vi "Create Dot.vi"(7 "3D Scatter Property":T4={"General Property"={"Plot Name"="", "Coordinate System"=enum."Cartesian", "Opacity"=0.0}, "Projection Property"={"Draw XY"=FALSE, "Draw YZ"=FALSE, "Draw XZ"=FALSE}, "Plot Property"={"Sprite Type"=enum."Empty Square", "Point Size"=0.0, "Color Ramp Cluster"={"Color Ramp Style"=enum."None", "Color Ramp Array"=[16711934, 393471, 57855, 4390754, 16449346, 16744722, 16711680], "Color Ramp Index"=[45, 91, 133, 175, 219, 255], "Interpolate?"=FALSE, "Logarithm?"=FALSE}}}, 8 "error in (no error)":errorcluster, 9 "Actual Transform In":T7, 10 "Plot Representation In":T1, 11 "Plot Object In":refnum<vi>) -> (0 "error out":errorcluster, 1 "Actual Transform Out":T7, 2 "Plot Representation Out":T1, 3 "Plot Object Out":refnum<vi>, 4 "Dot Object Out":refnum<vi>)   [LabVIEW 2020, in "3D Scatter.lvclass"]
uses:
  <vilib>/Math Plots/3D Math Plots/3D Scatter/3D Scatter/3D Scatter.lvclass
  <vilib>/Math Plots/3D Math Plots/3D Plot/3D Plot/Typedef/Actual Transform.ctl
  <vilib>/Math Plots/3D Math Plots/3D Plot/3D Plot/Typedef/Range Clusters.ctl
  <vilib>/Math Plots/3D Math Plots/3D Plot/3D Plot/Typedef/Plot Representation.ctl
  <vilib>/Math Plots/3D Math Plots/3D Plot/3D Plot/Typedef/Mesh Data.ctl
  <vilib>/Math Plots/3D Math Plots/3D Scatter/3D Scatter/Typedef/3D Scatter Property.ctl
  <vilib>/Math Plots/3D Math Plots/3D Plot/3D Plot/Typedef/Sprite Type.ctl
  <vilib>/Math Plots/3D Math Plots/3D Plot/3D Plot/Typedef/Color Ramp Cluster.ctl
  <vilib>/picture/3D Picture Control/NI_3D Picture Control.lvlib
  <vilib>/Math Plots/3D Math Plots/3D Plot/3D Plot/3D Plot.lvclass
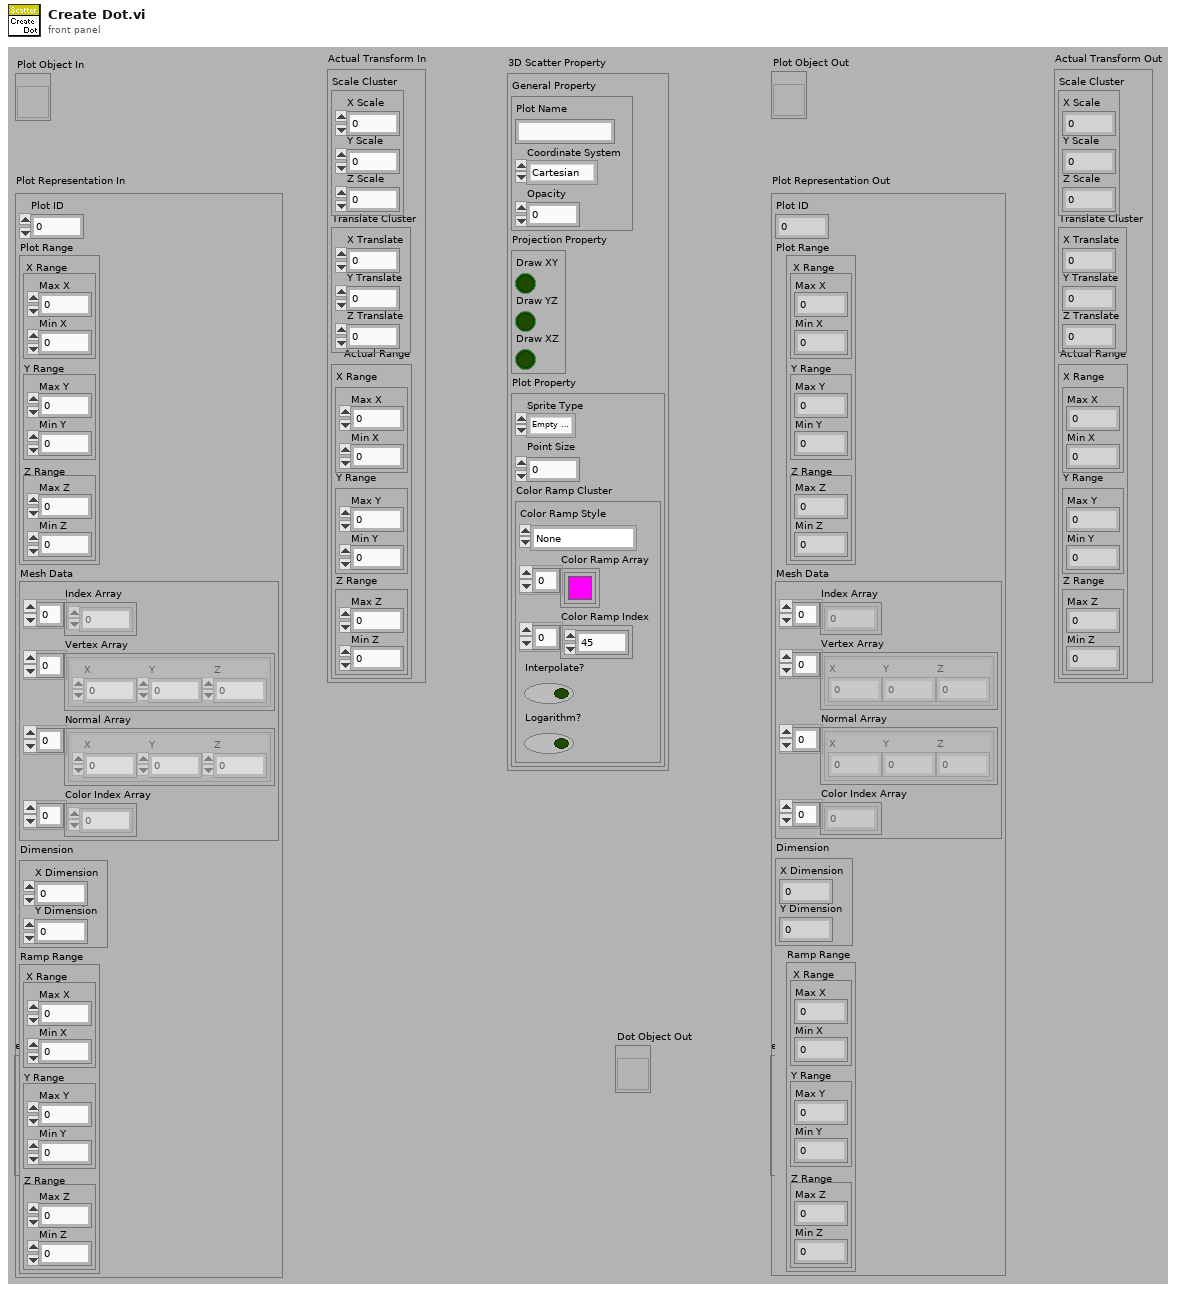
[diagram p1: front panel]
types:
  T1 = typedef "3D Plot.lvclass/Plot Representation.ctl" = cluster{"Plot ID":i32, "Plot Range":T2, "Mesh Data":T3, "Dimension":cluster{"X Dimension":i32, "Y Dimension":i32}, "Ramp Range":T2}
  T2 = typedef "3D Plot.lvclass/Range Clusters.ctl" = cluster{"X Range":cluster{"Max X":sgl, "Min X":sgl}, "Y Range":cluster{"Max Y":sgl, "Min Y":sgl}, "Z Range":cluster{"Max Z":sgl, "Min Z":sgl}}
  T3 = typedef "3D Plot.lvclass/Mesh Data.ctl" = cluster{"Index Array":u32[], "Vertex Array":cluster{"X":sgl, "Y":sgl, "Z":sgl}[], "Normal Array":cluster{"X":sgl, "Y":sgl, "Z":sgl}[], "Color Index Array":i32[]}
  T4 = typedef "3D Scatter.lvclass/3D Scatter Property.ctl" = cluster{"General Property":cluster{"Plot Name":string, "Coordinate System":enum16{"Cartesian", "Cylindrical", "Spherical"}, "Opacity":sgl}, "Projection Property":cluster{"Draw XY":bool, "Draw YZ":bool, "Draw XZ":bool}, "Plot Property":cluster{"Sprite Type":T5, "Point Size":sgl, "Color Ramp Cluster":T6}}
  T5 = typedef "3D Plot.lvclass/Sprite Type.ctl" = enum16{"None", "Empty Square", "Solid Square", "Empty Diamond", "Solid Diamond", "Empty Circle", "Solid Circle", "Asterisk", "Bold X", "Wireframe Sphere", "Solid Sphere", "Wireframe Cube", "Solid Cube"}
  T6 = typedef "3D Plot.lvclass/Color Ramp Cluster.ctl" = cluster{"Color Ramp Style":enum16{"None", "Shaded", "Color spectrum", "Grey scale", "Custom"}, "Color Ramp Array":u32[], "Color Ramp Index":i32[], "Interpolate?":bool, "Logarithm?":bool}
  T7 = typedef "3D Plot.lvclass/Actual Transform.ctl" = cluster{"Scale Cluster":cluster{"X Scale":sgl, "Y Scale":sgl, "Z Scale":sgl}, "Translate Cluster":cluster{"X Translate":sgl, "Y Translate":sgl, "Z Translate":sgl}, "Actual Range":T2}
  T8 = enum16{"Points", "Lines", "Line Strip", "Line Loop", "Triangles", "Triangle Strip", "Triangle Fan", "Quads", "Quad Strip", "Polygon"}
  T9 = enum16{"Overall", "Per Primitive", "Per Vertex", "Binding Off"}
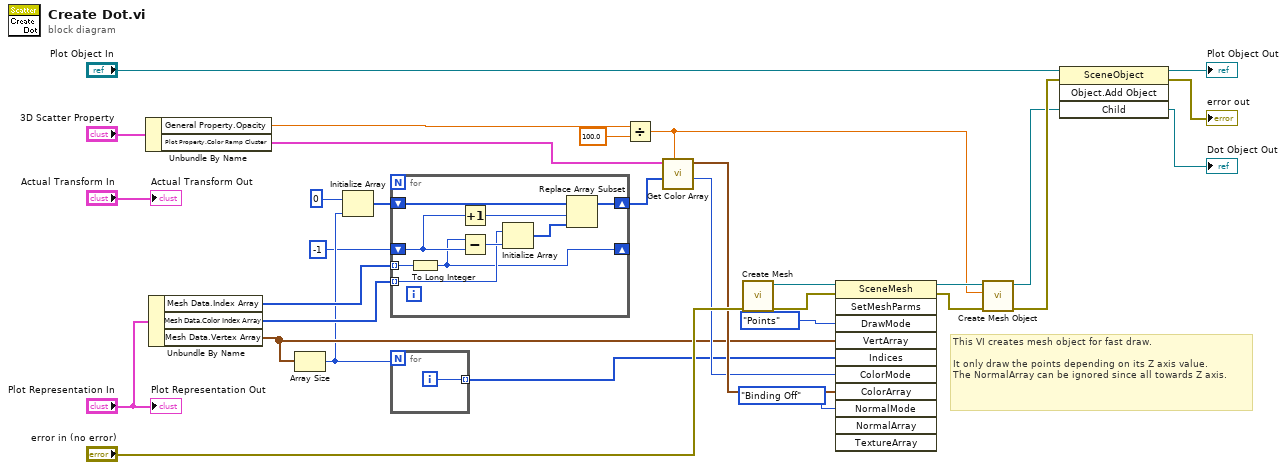
[diagram p0: block diagram]
diagram:
  # "This VI creates mesh object for fast draw.\n\nIt only draw the points depending on its Z axis value. \nThe NormalArray can be ignored since all towards Z axis."
  n1 = Unbundle By Name("3D Scatter Property") -> ("General Property.Opacity"=w24:sgl, "Plot Property.Color Ramp Cluster"=w10:T6)
  n2 = Unbundle By Name("Plot Representation In") -> ("Mesh Data.Index Array"=w8:u32[], "Mesh Data.Color Index Array"=w7:i32[], "Mesh Data.Vertex Array"=w6:cluster{"X":sgl, "Y":sgl, "Z":sgl}[])
  n3 = Array Size(array=w6) -> (size(s)=w5:i32)
  n4 = Initialize Array(0, w5) -> (w4:i32[])
  n5 = for {
    tunnel: w8 -> [w34] mode=indexing
    tunnel: w7 -> [w39] mode=indexing
    shift-right: [w37] -> w3
    shift-left: w4 -> [w38]
    shift-right: [w33] -> _
    shift-left: -1 -> [w35]
    n6 = To Long Integer(number=w34) -> (32bit integer=w33:i32)
    n7 = Increment(x=w35) -> (x+1=w32:i32)
    n8 = Subtract(x=w33, y=w35) -> (x-y=w40:i32)
    n9 = Initialize Array(w39, w40) -> (w36:i32[])
    n10 = Replace Array Subset(array=w38, new element=w36, index=w32) -> (w37:i32[])
  }
  n11 = for {
    N: w5 -> [_]
    tunnel: [w41] -> w9 mode=indexing
    i -> [w41]
  }
  n12 = Divide(x=w24, y=sgl 100.0) -> (x/y=w11:sgl)
  n13 = call <vilib>:"Get Color Array.vi"("Alpha"=w11, "Color Index Array"=w3, "Color Ramp Cluster"=w10) -> ("Color Binding Mode"=w18:T9, "Color Array"=w19:cluster{"R":sgl, "G":sgl, "B":sgl, "A":sgl}[])  [unwired: 4 in, 3 out]
  n14 = call <vilib>:"Create Mesh.vi"("error in (no error)"="error in (no error)") -> ("error out"=w21:errorcluster, "New Mesh Refnum"=w23:refnum<vi>)  [unwired: 9 out]
  n15 = invoke class="SceneMesh" method="SetMeshParms"(reference=w23, error in=w21, "DrawMode"=T8."Points" ("Draw Mode"), "VertArray"=w6, "Indices"=w9, "ColorMode"=w18, "ColorArray"=w19, "NormalMode"=T9."Binding Off" ("Normal Binding Mode")) -> (reference out=w15:refnum<vi>, error out=w14:errorcluster)  [unwired: 3 in, 9 out]
  n16 = call <vilib>:"Create Mesh Object.vi"("error in (no error)"=w14, "Alpha"=w11, "Mesh Object In"=w15) -> ("error out"=w13:errorcluster, "Object Ref Out"=w12:refnum<vi>)  [unwired: 1 in, 6 out]
  n17 = invoke class="SceneObject" method="Object.Add Object"(reference="Plot Object In", error in=w13, "Child"=w12) -> (reference out=→"Plot Object Out":refnum<vi>, error out=→"error out":errorcluster, "Child"=→"Dot Object Out":refnum<vi>)  [unwired: 1 in, 1 out]
  "Actual Transform Out" <- "Actual Transform In"
  "Plot Representation Out" <- "Plot Representation In"
